vi "Destroy.vi"(8 "error in":errorcluster, 11 "Gluing Procedure in":refnum<class "Gluing Procedure.lvclass">) -> (0 "error out":errorcluster)   [LabVIEW 2011, in "Gluing Procedure.lvclass"]
uses:
  Gluing Procedure.lvclass
  Gluing Procedure.lvclass/Gluing Procedure.ctl
  Shared Components/Gantry Class/Gantry Class.lvclass
  Shared Components/Config Manager Class/Config Manager Class.lvclass
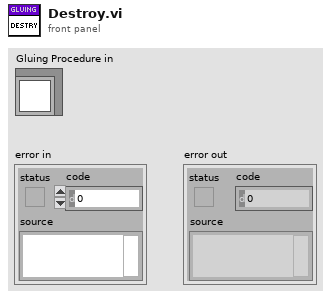
[diagram p1: front panel]
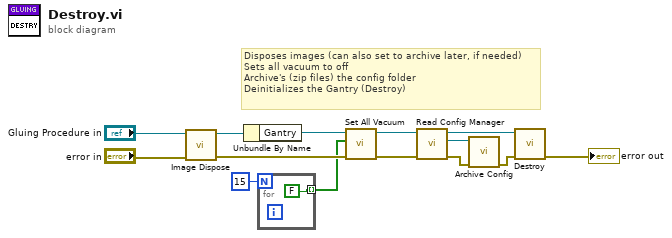
[diagram p0: block diagram]
diagram:
  # "Disposes images (can also set to archive later, if needed)\nSets all vacuum to off\nArchive's (zip files) the config folder\nDeinitializes the Gantry (Destroy)"
  n1 = call "Image Dispose.vi"("error in"="error in", "Gluing Procedure in"="Gluing Procedure in") -> ("error out"=w4:errorcluster, "Gluing Procedure out"=w5:refnum<class "Gluing Procedure.lvclass">)  [unwired: 8 in]
  n2 = Unbundle By Name(w5) -> ("Gantry"=w8:refnum<class "Gantry Class.lvclass">)
  n3 = for {
    N: 15 -> [_]
    tunnel: [FALSE] -> w2 mode=indexing
  }
  n4 = call "Set All Vacuum.vi"("error in"=w4, "Channel Array"=w2, "Gantry Class in"=w8) -> ("error out"=w7:errorcluster, "Gantry Class out"=w9:refnum<class "Gantry Class.lvclass">)  [unwired: 7 in]
  n5 = call-dynamic "Read Config Manager.vi"("error in"=w7, "Gantry in"=w9) -> ("error out"=w13:errorcluster, "Config Manager"=w14:refnum<class "Config Manager Class.lvclass">, "Gantry out"=w12:refnum<class "Gantry Class.lvclass">)  [unwired: 7 in]
  n6 = call "Archive Config.vi"("error in"=w13, "Config Manager in"=w14) -> ("error out"=w11:errorcluster)  [unwired: 8 in, 1 out]
  n7 = call "Destroy.vi"("error in"=w11, "Gantry Class in"=w12) -> ("error out"=→"error out":errorcluster)  [unwired: 9 in]
